vi "Client.vi"() -> ()   [LabVIEW 2021]
panel:
  out "Iteration":i32
  out "Random Number Received":dbl
  in  "data in":string="15 50 20 30 50"
  out "error out":errorcluster
  in  "stop":bool
  out "String":string
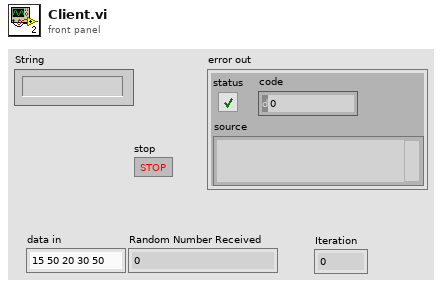
[diagram p1: front panel]
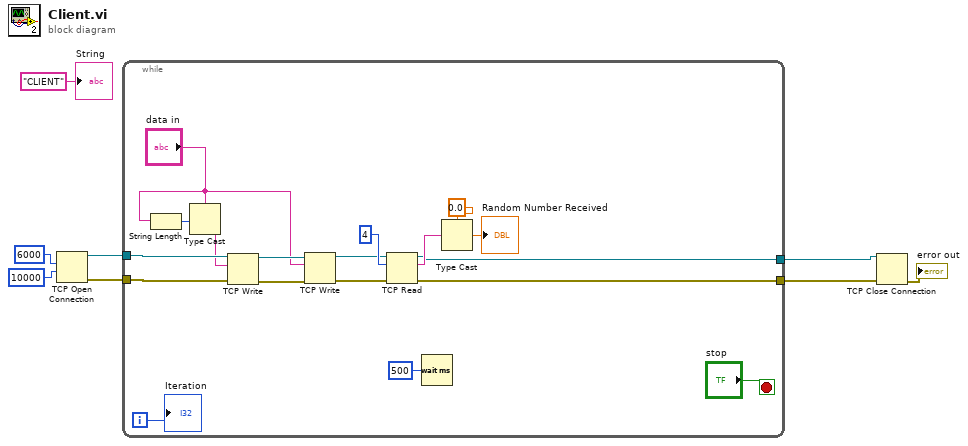
[diagram p0: block diagram]
diagram:
  n1 = TCP Open Connection(remote port or service name=u16 6000 ("port"), timeout ms (60000)=10000 ("timeout ms (wait forever: -1)")) -> (connection ID=w2:refnum<k5>, error out=w3:errorcluster)  [unwired: 3 in]
  n2 = while {
    tunnel: [w11] -> w7
    tunnel: w3 -> [w24]
    tunnel: w2 -> [w23]
    tunnel: [w10] -> w1
    i -> [w18]
    stop <- "stop" stop-if-true
    n3 = String Length(string="data in") -> (length=w25:i32)
    n4 = Type Cast(type="data in", x=w25) -> (*(type *) &x=w20:string)
    n5 = TCP Write(connection ID=w23, data in=w20, error in (no error)=w24) -> (connection ID out=w21:refnum<k5>, error out=w22:errorcluster)  [unwired: 1 in, 1 out]
    n6 = TCP Write(connection ID=w21, data in="data in", error in (no error)=w22) -> (connection ID out=w12:refnum<k5>, error out=w14:errorcluster)  [unwired: 1 in, 1 out]
    n7 = TCP Read(connection ID=w12, bytes to read=4, error in (no error)=w14) -> (connection ID out=w10:refnum<k5>, data out=w16:string, error out=w11:errorcluster)  [unwired: 2 in]
    n8 = Wait (ms)(milliseconds to wait=u32 500) -> ()  [unwired: 1 out]
    n9 = Type Cast(type=0.0, x=w16) -> (*(type *) &x=→"Random Number Received":dbl)
    "Iteration" <- w18
  }
  n10 = TCP Close Connection(connection ID=w1, error in (no error)=w7) -> (error out=→"error out":errorcluster)  [unwired: 1 in, 1 out]
  "String" <- "CLIENT" ("String")
